vi "Fault_ID_Parse.vi"(8 "Enum":enum16{"Sequence", "Table"}(ring), 11 "Numeric":u32) -> (3 "String":string)   [LabVIEW 2016]
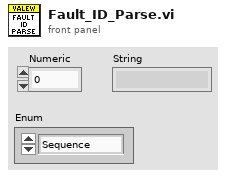
[diagram p1: front panel]
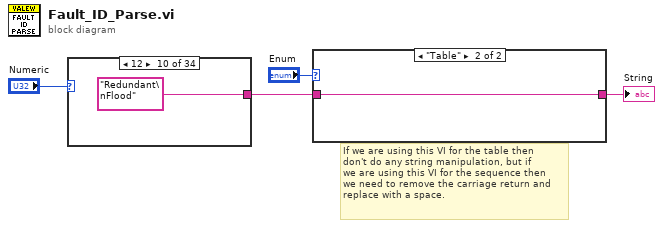
[diagram p0: block diagram]
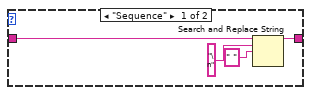
[diagram p2: hidden frame]
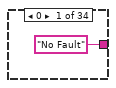
[diagram p3: hidden frame]
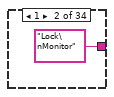
[diagram p4: hidden frame]
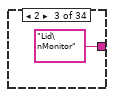
[diagram p5: hidden frame]
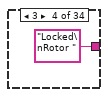
[diagram p6: hidden frame]
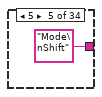
[diagram p7: hidden frame]
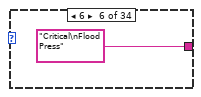
[diagram p8: hidden frame]
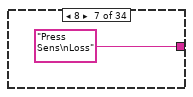
[diagram p9: hidden frame]
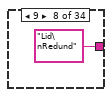
[diagram p10: hidden frame]
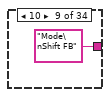
[diagram p11: hidden frame]
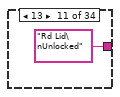
[diagram p12: hidden frame]
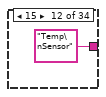
[diagram p13: hidden frame]
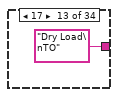
[diagram p14: hidden frame]
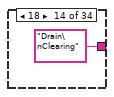
[diagram p15: hidden frame]
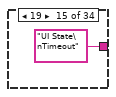
[diagram p16: hidden frame]
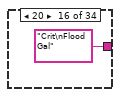
[diagram p17: hidden frame]
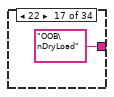
[diagram p18: hidden frame]
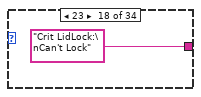
[diagram p19: hidden frame]
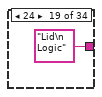
[diagram p20: hidden frame]
diagram:
  # "If we are using this VI for the table then\ndon't do any string manipulation, but if\nwe are using this VI for the sequence then\nwe need to remove the carriage return and\nreplace with a space."
  n1 = case shown="12" "Numeric" {
    selector: "Numeric" -> [_ _ _ _ _ _ _ _ _ _ _ _ _ _ _ _ _ _ _ _ _ _ _ _ _ _ _ _ _ _ _ _ _ w39]
    tunnel: ["No Fault" "Lock\nMonitor" "Lid\nMonitor" "Locked\nRotor " "Mode\nShift" "Critical\nFlood Press" "Press Sens\nLoss" "Lid\nRedund" "Mode\nShift FB" "Redundant\nFlood" "Rd Lid\nUnlocked" "Temp\nSensor" "Dry Load\nTO" "Drain\nClearing" "UI State\nTimeout" "Crit\nFlood Gal" "OOB\nDryLoad" "Crit LidLock:\nCan't Lock" "Lid\n Logic" "Press Sens\nDropout" "OOB\nRedist" "Water\nAccess" "ADC \nKnob" "Suds\nLock" "Stuck\nButton" "OOB\nFallback" "Crit LidLock:\nCan't Unlock" "Accelrmtr\nComm" "Flood\nWarning" "Clock\nMon" "LidLock\nFailure" "Adaptive\nDrain" "Flood\nWarn Gal" w38] -> w3
    frame 0 {
    }
    frame 1 {
    }
    frame 2 {
    }
    frame 3 {
    }
    frame 5 {
    }
    frame 6 {
    }
    frame 8 {
    }
    frame 9 {
    }
    frame 10 {
    }
    frame 12 {
    }
    frame 13 {
    }
    frame 15 {
    }
    frame 17 {
    }
    frame 18 {
    }
    frame 19 {
    }
    frame 20 {
    }
    frame 22 {
    }
    frame 23 {
    }
    frame 24 {
    }
    frame 25 {
    }
    frame 26 {
    }
    frame 27 {
    }
    frame 28 {
    }
    frame 29 {
    }
    frame 30 {
    }
    frame 31 {
    }
    frame 32 {
    }
    frame 100 {
    }
    frame 101 {
    }
    frame 102 {
    }
    frame 103 {
    }
    frame 104 {
    }
    frame 105 {
    }
    frame Default {
      n2 = Number To Decimal String(number=w39) -> (decimal integer string=w38:string)  [unwired: 1 in]
    }
  }
  n3 = case shown="\"Table\"" "Enum" {
    tunnel: w3 -> [w43 w44]
    tunnel: [w40 w44] -> w2
    frame "Sequence" {
      n4 = Search and Replace String(input string=w43, search string="\n", replace string=" " ("replace string (\"\")")) -> (result string=w40:string)  [unwired: 5 in, 3 out]
    }
    frame "Table" {
    }
  }
  "String" <- w2
